vi "Labview5_2.vi"() -> ()   [LabVIEW 2019]
panel:
  out "Waveform Graph":dbl[](graph)
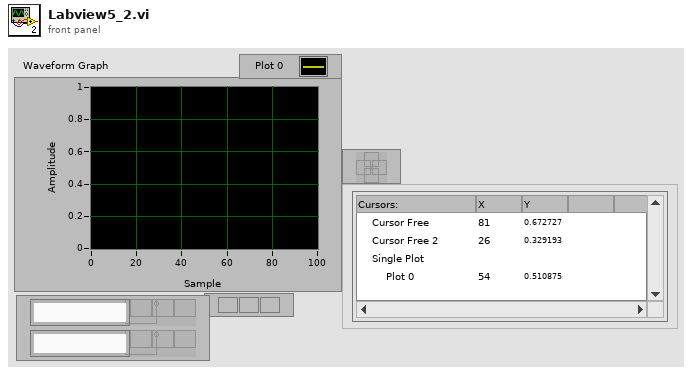
[diagram p1: front panel]
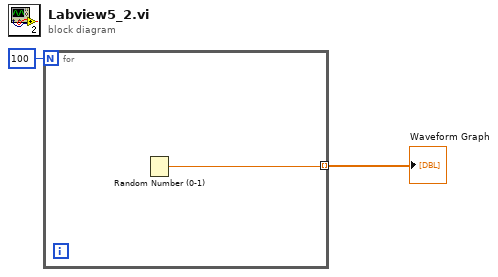
[diagram p0: block diagram]
diagram:
  n1 = for {
    N: 100 -> [_]
    tunnel: [w3] -> w1 mode=indexing
    n2 = Random Number (0-1)() -> (number: 0 to 1=w3:dbl)
  }
  "Waveform Graph" <- w1
